vi "Get Discovery Info.vi"(8 "error in (no error)":errorcluster, 11 "Node in":refnum<class "Node Config.lvclass">) -> (0 "error out":errorcluster, 2 "Discovery Info":T1, 3 "Node out":refnum<class "Node Config.lvclass">)   [LabVIEW 2020, in "Vecto.lvlib" / "Node Config.lvclass"]
uses:
  Node Config.lvclass
  Discovery Info.ctl
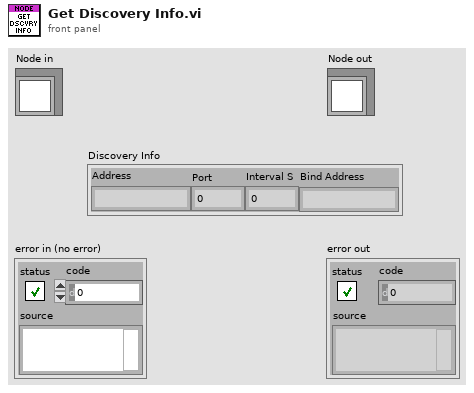
[diagram p1: front panel]
types:
  T1 = typedef "Vecto.lvlib/Node Config.lvclass/Discovery Info.ctl" = cluster{"Address":string, "Port":u16, "Interval S":dbl, "Bind Address":string}
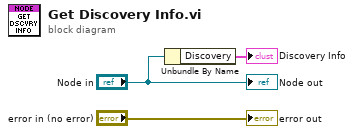
[diagram p0: block diagram]
diagram:
  n1 = Unbundle By Name("Node in") -> ("Discovery"=→"Discovery Info":T1)
  "error out" <- "error in (no error)"
  "Node out" <- "Node in"
